vi "Main.vi"() -> ()   [LabVIEW 2020, in "S7.lvlib"]
doc: "This template is based off of the Queued Message Handler design pattern and the Queued Message Handler project template that ships with LabVIEW.\n\nThe main difference is that the queue is private to this module and communication between modules is performed via Broadcast and Request events.\n\nRequest events are wrapped in public API methods and are handled in the Event Handling Loop (EHL) of this VI. Any module can register for Broadcast events sent by this module. The EHL generates messages based on user interface actions.\n\nThe Message Handling Loop (MHL) processes messages generated by the EHL, or by other messages. The messages are string values, so new messages can be added easily to the Message Cases case structure in the MHL. Each message cluster can also provide an optional value for Message Data, which is a variant that can be converted to whatever message-specific data is required.\n_____\nBased on Delacor QMH Project Template 4.1.0.59."
uses:
  S7.lvlib
  <vilib>/Delacor/Delacor QMH/Libraries/Module Admin_class/Delacor_lib_QMH_Module Admin.lvclass
  Module Data--cluster.ctl
  <vilib>/Delacor/Delacor QMH/Libraries/Message Queue_class/Delacor_lib_QMH_Message Queue.lvclass/Delacor_lib_QMH_Message Queue.ctl
  Stop Argument--cluster.ctl
  <vilib>/Delacor/Delacor QMH/Libraries/Module Admin_class/Delacor_lib_QMH_Module Admin.lvclass/Delacor_lib_QMH_Module Admin.ctl
  Init S7 Link Argument--cluster.ctl
  Close S7 Link Argument--cluster.ctl
  Read_Data Argument--cluster.ctl
  Read_Data (Reply Payload)--cluster.ctl
  Write_Data Argument--cluster.ctl
  Write_Data (Reply Payload)--cluster.ctl
  <vilib>/Utility/miscctls.llb/LVPointTypeDef.ctl
  <vilib>/Delacor/Delacor QMH/Libraries/Message Queue_class/Delacor_lib_QMH_Enqueue Message (Single).vi
  <vilib>/Delacor/Delacor QMH/Libraries/Module Admin_class/Delacor_lib_QMH_Get External Launch.vi
  <vilib>/Utility/error.llb/Error Cluster From Error Code.vi
  <vilib>/ErrorRing/Error Ring.xnode
  <vilib>/Delacor/Delacor QMH/Libraries/Message Queue_class/Delacor_lib_QMH_Message Queue.lvclass
panel:
  out "S7 Link":refnum<k5>
  in  "Simulate MHL Error":bool
  in  "Simulate EHL Error":bool
  out "error out":errorcluster
  in  "Module Admin":refnum<class "Delacor_lib_QMH_Module Admin.lvclass">
  out "Status":string
  # "Other QMH Modules communicate with this Module via its Public API (wrappers for its Request Events).\n\nThis Module communicates with other Modules via its Broadcast Events.\nAny module that wants to get these messages, just registers for this module's Broadcast events."
  # "This template is for the Delacor Modified Queued Message Handler design pattern.\n\nSee the block diagram for more information on how to use this template."
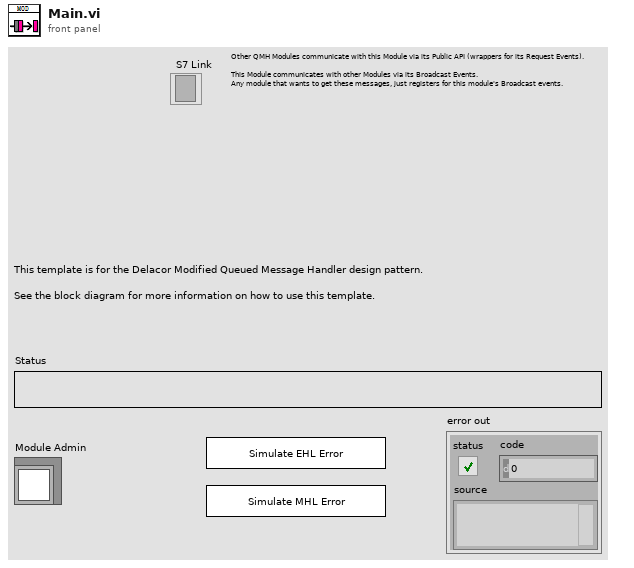
[diagram p1: front panel]
types:
  T1 = typedef "S7.lvlib/Request Events--cluster.ctl" = cluster{"Stop Module":refnum<user-event>, "Show Panel":refnum<user-event>, "Hide Panel":refnum<user-event>, "Get Module Execution Status":refnum<user-event>, "Show Diagram":refnum<user-event>, "S7_Open":refnum<user-event>, "Init S7 Link":refnum<user-event>, "Close S7 Link":refnum<user-event>, "Read_Data":refnum<user-event>, "Write_Data":refnum<user-event>}
  T2 = typedef "S7.lvlib/Module Data--cluster.ctl" = cluster{"Status":string}
  T3 = enum32{"invalid lock state", "Not Locked", "Locked (No Password)", "Password-protected"}
  T4 = typedef "S7.lvlib/Stop Argument--cluster.ctl" = cluster{"Origin":string, "Exit via Stop Module Req?":bool, "Wait for Module to stop?":bool}
  T5 = typedef "S7.lvlib/Init S7 Link Argument--cluster.ctl" = cluster{"IP":string, "超时":i32}
  T6 = typedef "S7.lvlib/Close S7 Link Argument--cluster.ctl" = cluster{"布尔":bool}
  T7 = typedef "S7.lvlib/Read_Data Argument--cluster.ctl" = cluster{"DB #":u16, "起始地址":u32, "寄存器类型":u8, "读取长度":u16, "数据类型":u16, "Wait Notifier":refnum<notifier>, "wait for reply":bool}
  T8 = typedef "S7.lvlib/Write_Data Argument--cluster.ctl" = cluster{"写入数据":u32, "DB #":u16, "写入地址":u32, "寄存器类型":u8, "数据类型":u16, "Wait Notifier":refnum<notifier>, "wait for reply":bool}
  T9 = typedef "LVPointTypeDef.ctl" = cluster{"Horizontal":i16, "Vertical":i16}
  T10 = enum32{"Invalid", "Standard", "Closed", "Hidden", "Minimized", "Maximized"}
  T11 = typedef "S7.lvlib/Read_Data (Reply Payload)--cluster.ctl" = cluster{"读取成功":bool, "数据":u32[], "Read_Data_error":errorcluster}
  T12 = typedef "S7.lvlib/Write_Data (Reply Payload)--cluster.ctl" = cluster{"写入成功":bool, "Write_Data_error":errorcluster}
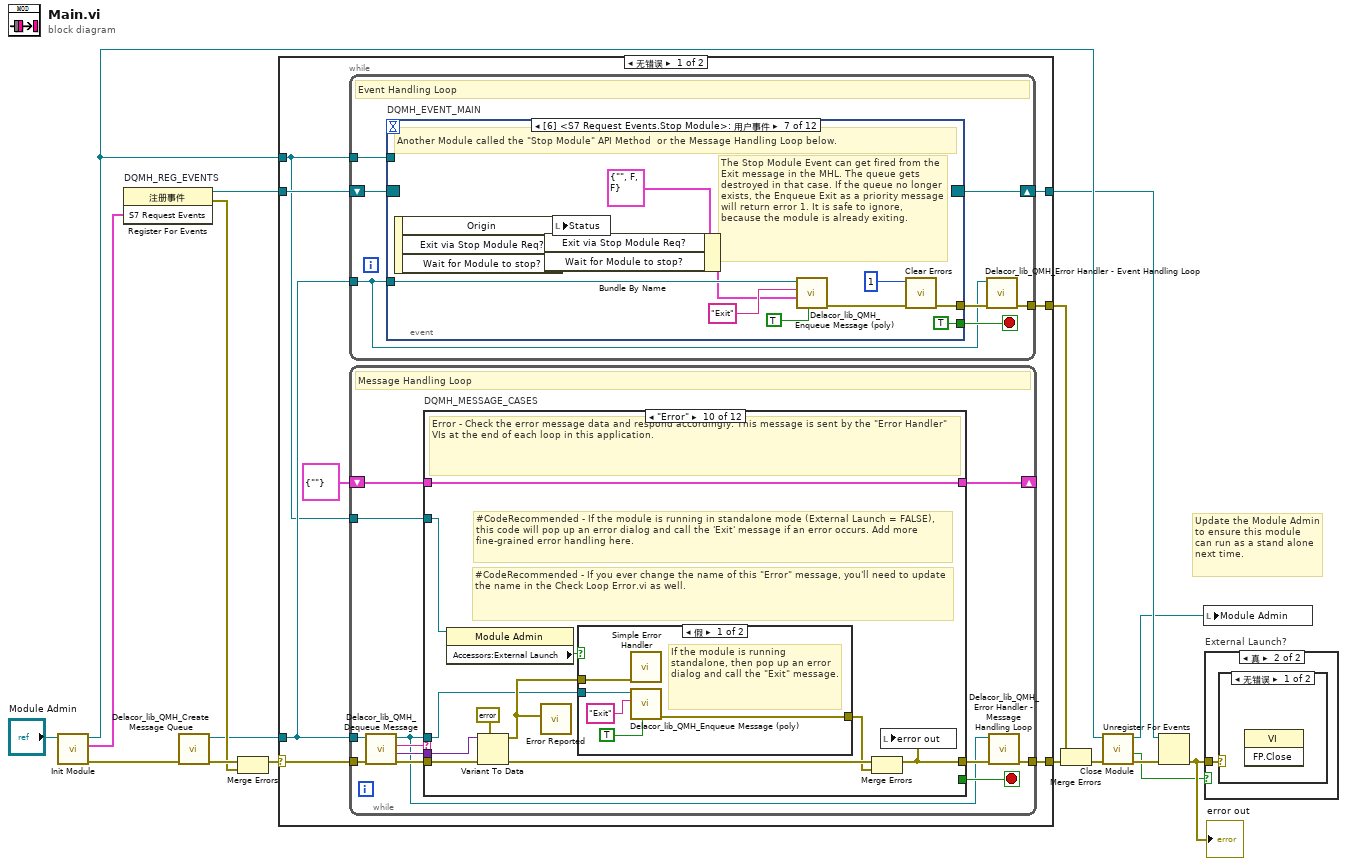
[diagram p0: block diagram]
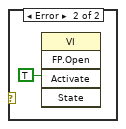
[diagram p3: hidden frame]
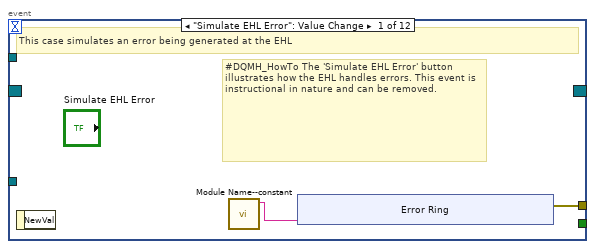
[diagram p4: hidden frame]
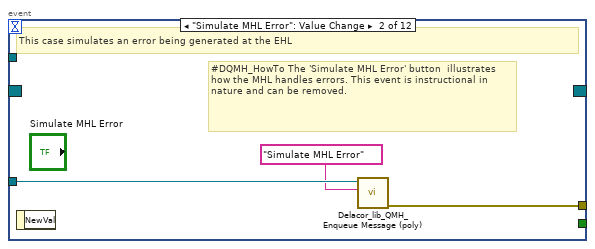
[diagram p5: hidden frame]
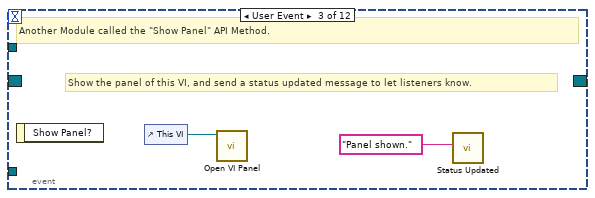
[diagram p6: hidden frame]
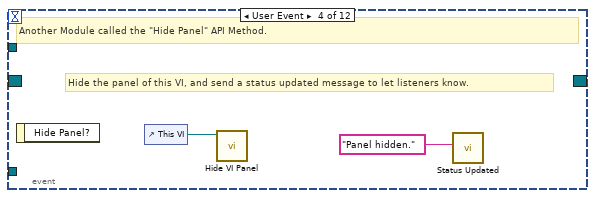
[diagram p7: hidden frame]
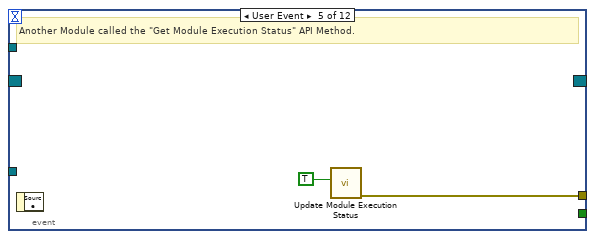
[diagram p8: hidden frame]
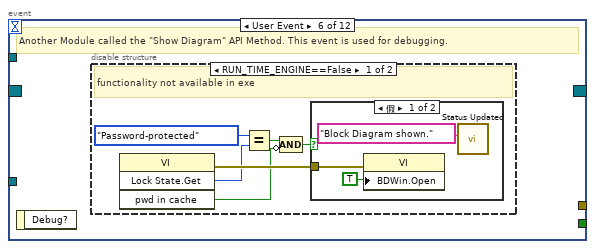
[diagram p9: hidden frame]
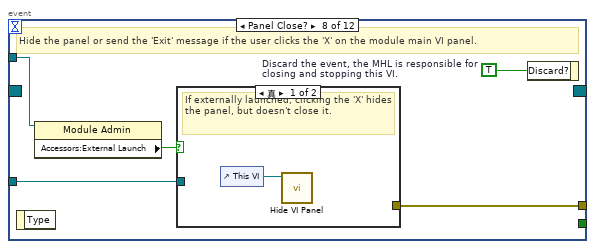
[diagram p12: hidden frame]
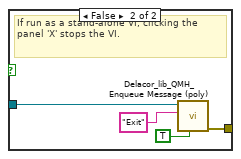
[diagram p13: hidden frame]
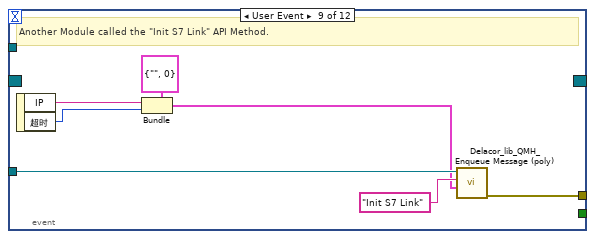
[diagram p14: hidden frame]
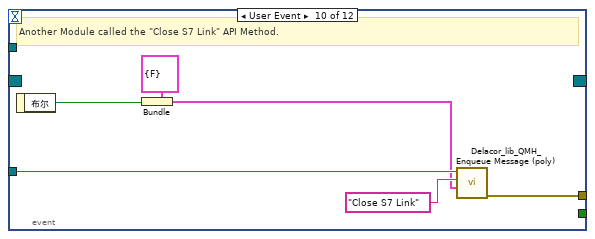
[diagram p15: hidden frame]
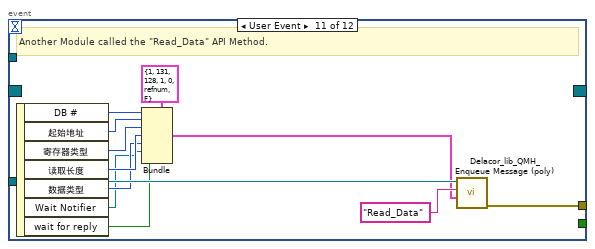
[diagram p16: hidden frame]
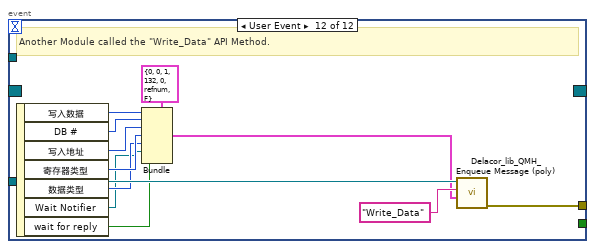
[diagram p17: hidden frame]
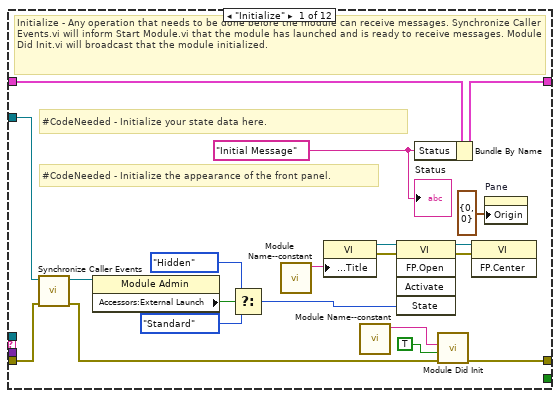
[diagram p18: hidden frame]
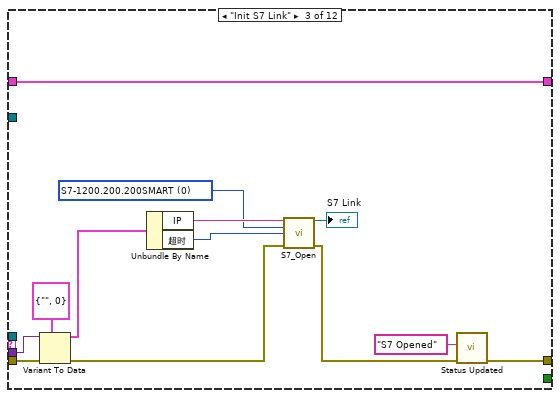
[diagram p20: hidden frame]
diagram:
  # "Update the Module Admin to ensure this module can run as a stand alone next time."
  n1 = call "Init Module.vi"("Singleton Module Admin in"="Module Admin") -> ("error out"=w16:errorcluster, "S7 Request Events"=w5:T1, "Singleton Module Admin out"=w8:refnum<class "Delacor_lib_QMH_Module Admin.lvclass">)  [unwired: 8 in]
  n2 = register-events "DQMH_REG_EVENTS"(w5) -> (reference out=w6:refnum<event-registration>, error out=w9:errorcluster)  [unwired: 2 in]
  n3 = call <vilib>:"Delacor_lib_QMH_Create Message Queue.vi"("error in"=w16) -> ("error out"=w11:errorcluster, "Message Queue"=w4:refnum<class "Delacor_lib_QMH_Message Queue.lvclass">)  [unwired: 9 in]
  n4 = Merge Errors(w11, w9) -> (w10:errorcluster)
  n5 = case shown="无错误" w10 {
    selector: w10 -> [w23 w290]
    tunnel: [w25 w290] -> w17
    tunnel: [w22 w287] -> w7
    tunnel: w6 -> [w20 w287]
    tunnel: w4 -> [w19 _]
    tunnel: [w24 _] -> w14
    tunnel: w8 -> [w18 w283]
    frame No Error {
      n6 = while {
        tunnel: w19 -> [w26]
        shift-right: [w29] -> w22
        shift-left: w20 -> [w30]
        tunnel: [w31] -> w24
        tunnel: w18 -> [w27]
        stop <- w28 stop-if-true
        # "Event Handling Loop"
        n7 = event "DQMH_EVENT_MAIN" shown="[6] <S7 Request Events.Stop Module>: 用户事件" {
          selector: w30 -> [_ _ _ _ _ _ _ _ _ _ _ _]
          dyn-events: [_ _ _ _ _ _ _ _ _ _ _ _] -> w29
          timeout: _ -> [_ _ _ _ _ _ _ _ _ _ _ _]
          tunnel: [_ _ _ _ _ _ TRUE ("Discard?") _ _ _ _ _] -> w28
          tunnel: w26 -> [_ w43 _ _ _ _ w67 w74 w88 w94 w106 w118]
          tunnel: [w34 w44 _ _ w50 _ w70 w76 w82 w89 w95 w107] -> w32
          tunnel: w27 -> [_ _ _ _ _ _ _ w73 _ _ _ _]
          event "Simulate EHL Error": Value Change {
            # "#DQMH_HowTo The 'Simulate EHL Error' button  illustrates how the EHL handles errors. This event is instructional in nature and can be removed."
            # "This case simulates an error being generated at the EHL"
            n8 = event-data() -> ()  [unwired: 1 in, 1 out]
            n9 = call "Module Name--constant.vi"() -> ("Module Name"=w33:string)  [unwired: 11 in]
            n10 = xnode "Error Ring"("参数 0"=w33) -> ("错误输出"=w34:errorcluster)
          }
          event "Simulate MHL Error": Value Change {
            # "#DQMH_HowTo The 'Simulate MHL Error' button  illustrates how the MHL handles errors. This event is instructional in nature and can be removed."
            # "This case simulates an error being generated at the EHL"
            n11 = event-data() -> ()  [unwired: 1 in, 1 out]
            n12 = call-poly <vilib>:"Delacor_lib_QMH_Enqueue Message (poly).vi"("Message"="Simulate MHL Error", "Message Queue in"=w43) -> ("error out"=w44:errorcluster)  [unwired: 8 in, 1 out]
          }
          event User Event {
            # "Show the panel of this VI, and send a status updated message to let listeners know."
            # "Another Module called the \"Show Panel\" API Method."
            n13 = event-data() -> ()  [unwired: 1 in, 1 out]
            n14 = control-ref of="This VI"() -> (w46:refnum<vi>)
            n15 = call "Open VI Panel.vi"("VI"=w46) -> ()  [unwired: 10 in, 1 out]
            n16 = call "Status Updated.vi"("Status"="Panel shown." ("format string")) -> ()  [unwired: 10 in, 1 out]
          }
          event User Event {
            # "Hide the panel of this VI, and send a status updated message to let listeners know."
            # "Another Module called the \"Hide Panel\" API Method."
            n17 = event-data() -> ()  [unwired: 1 in, 1 out]
            n18 = control-ref of="This VI"() -> (w48:refnum<vi>)
            n19 = call "Hide VI Panel.vi"("VI"=w48) -> ()  [unwired: 10 in, 1 out]
            n20 = call "Status Updated.vi"("Status"="Panel hidden." ("format string")) -> ()  [unwired: 10 in, 1 out]
          }
          event User Event {
            # "Another Module called the \"Get Module Execution Status\" API Method."
            n21 = event-data() -> ()  [unwired: 1 in, 1 out]
            n22 = call "Update Module Execution Status.vi"("Running?"=TRUE) -> ("error out"=w50:errorcluster)  [unwired: 10 in]
          }
          event User Event {
            # "Another Module called the \"Show Diagram\" API Method. This event is used for debugging."
            n23 = event-data() -> ()  [unwired: 1 in, 1 out]
            n24 = disable-structure shown="RUN_TIME_ENGINE==False" {
              frame condition #0 (active) {
                # "functionality not available in exe"
                n25 = invoke class="VI" method="Lock State.Get"() -> (error out=w56:errorcluster, "Get Lock State"=w55:T3, "pwd in cache"=w52:bool)  [unwired: 4 in, 1 out]
                n26 = Equal?(x=T3."Password-protected", y=w55) -> (x = y?=w53:bool)
                n27 = Compound Arithmetic op=AND(w53, invert w52) -> (w51:bool)
                n28 = case "条件结构" shown="假" w51 {
                  tunnel: w56 -> [w59 _]
                  frame False {
                    n29 = property class="VI"(error in=w59, "BDWin.Open"=TRUE ("Block Diagram Window:Open")) -> ()  [unwired: 1 in, 2 out]
                    n30 = call "Status Updated.vi"("Status"="Block Diagram shown." ("format string")) -> ()  [unwired: 10 in, 1 out]
                  }
                  frame True {
                    # "Password-protected VI, and the password is not in the cache. Do not show the diagram."
                  }
                }
              }
              frame condition #1 {
              }
            }
          }
          event User Event {
            # "The Stop Module Event can get fired from the Exit message in the MHL. The queue gets destroyed in that case. If the queue no longer exists, the Enqueue Exit as a priority message will return error 1. It is safe to ignore, because the module is already exiting."
            # "Another Module called the \"Stop Module\" API Method  or the Message Handling Loop below."
            n31 = event-data() -> ("Origin"=w66:string, "Exit via Stop Module Req?"=w62:bool, "Wait for Module to stop?"=w61:bool)  [unwired: 1 in]
            n32 = Bundle By Name(cluster=T4 {"Origin"="", "Exit via Stop Module Req?"=FALSE, "Wait for Module to stop?"=FALSE} ("Stop Argument"), "Exit via Stop Module Req?"=w62, "Wait for Module to stop?"=w61) -> (w60:T4)
            n33 = local write "Status"(w66) -> ()
            n34 = call-poly <vilib>:"Delacor_lib_QMH_Enqueue Message (poly).vi"("Priority Message? (F)"=TRUE, "Message Data"=w60, "Message"="Exit", "Message Queue in"=w67) -> ("error out"=w71:errorcluster)  [unwired: 6 in, 1 out]
            n35 = call <vilib>:"Clear Errors.vi"("error in (no error)"=w71, "specific error code to clear (0: all)"=1) -> ("error out"=w70:errorcluster)  [unwired: 4 in, 1 out]
          }
          event Panel Close? {
            w75 = TRUE  # Discard the event, the MHL is responsible for closing and stopping this VI.
            # "Hide the panel or send the 'Exit' message if the user clicks the 'X' on the module main VI panel."
            n36 = event-data() -> ()  [unwired: 1 in, 1 out]
            n37 = property class="Module Admin"(reference=w73) -> ("Accessors:External Launch"=w72:bool)  [unwired: 1 in, 2 out]
            n38 = case "条件结构" shown="真" w72 {
              tunnel: w74 -> [_ w80]
              tunnel: [_ w81] -> w76
              frame True {
                # "If externally launched, clicking the 'X' hides the panel, but doesn't close it."
                n39 = control-ref of="This VI"() -> (w77:refnum<vi>)
                n40 = call "Hide VI Panel.vi"("VI"=w77) -> ()  [unwired: 10 in, 1 out]
              }
              frame False {
                # "If run as a stand-alone VI, clicking the panel 'X' stops the VI."
                n41 = call-poly <vilib>:"Delacor_lib_QMH_Enqueue Message (poly).vi"("Priority Message? (F)"=TRUE, "Message"="Exit", "Message Queue in"=w80) -> ("error out"=w81:errorcluster)  [unwired: 7 in, 1 out]
              }
            }
            n42 = event-data("Discard?"=w75) -> ()  [unwired: 1 in, 1 out]
          }
          event User Event {
            # "Another Module called the \"Init S7 Link\" API Method."
            n43 = event-data() -> ("IP"=w84:string, "超时"=w83:i32)  [unwired: 1 in]
            n44 = Bundle(cluster=T5 {"IP"="", "超时"=0} ("Init S7 Link Argument"), "IP"=w84, "超时"=w83) -> (w85:T5)
            n45 = call-poly <vilib>:"Delacor_lib_QMH_Enqueue Message (poly).vi"("Message Data"=w85, "Message"="Init S7 Link", "Message Queue in"=w88) -> ("error out"=w82:errorcluster)  [unwired: 7 in, 1 out]
          }
          event User Event {
            # "Another Module called the \"Close S7 Link\" API Method."
            n46 = event-data() -> ("布尔"=w90:bool)  [unwired: 1 in]
            n47 = Bundle(cluster=T6 {"布尔"=FALSE} ("Close S7 Link Argument"), "布尔"=w90) -> (w91:T6)
            n48 = call-poly <vilib>:"Delacor_lib_QMH_Enqueue Message (poly).vi"("Message Data"=w91, "Message"="Close S7 Link", "Message Queue in"=w94) -> ("error out"=w89:errorcluster)  [unwired: 7 in, 1 out]
          }
          event User Event {
            # "Another Module called the \"Read_Data\" API Method."
            n49 = event-data() -> ("DB #"=w102:u16, "起始地址"=w101:u32, "寄存器类型"=w100:u8, "读取长度"=w99:u16, "数据类型"=w98:u16, "Wait Notifier"=w97:refnum<notifier>, "wait for reply"=w96:bool)  [unwired: 1 in]
            n50 = Bundle(cluster=T7 {"DB #"=1, "起始地址"=131, "寄存器类型"=128, "读取长度"=1, "数据类型"=0, "Wait Notifier"=refnum, "wait for reply"=FALSE} ("Read_Data Argument"), "DB #"=w102, "起始地址"=w101, "寄存器类型"=w100, "读取长度"=w99, "数据类型"=w98, "Wait Notifier"=w97, "wait for reply"=w96) -> (w103:T7)
            n51 = call-poly <vilib>:"Delacor_lib_QMH_Enqueue Message (poly).vi"("Message Data"=w103, "Message"="Read_Data", "Message Queue in"=w106) -> ("error out"=w95:errorcluster)  [unwired: 7 in, 1 out]
          }
          event User Event {
            # "Another Module called the \"Write_Data\" API Method."
            n52 = event-data() -> ("写入数据"=w114:u32, "DB #"=w113:u16, "写入地址"=w112:u32, "寄存器类型"=w111:u8, "数据类型"=w110:u16, "Wait Notifier"=w109:refnum<notifier>, "wait for reply"=w108:bool)  [unwired: 1 in]
            n53 = Bundle(cluster=T8 {"写入数据"=0, "DB #"=0, "写入地址"=1, "寄存器类型"=132, "数据类型"=0, "Wait Notifier"=refnum, "wait for reply"=FALSE} ("Write_Data Argument"), "写入数据"=w114, "DB #"=w113, "写入地址"=w112, "寄存器类型"=w111, "数据类型"=w110, "Wait Notifier"=w109, "wait for reply"=w108) -> (w115:T8)
            n54 = call-poly <vilib>:"Delacor_lib_QMH_Enqueue Message (poly).vi"("Message Data"=w115, "Message"="Write_Data", "Message Queue in"=w118) -> ("error out"=w107:errorcluster)  [unwired: 7 in, 1 out]
          }
        }
        n55 = call-dynamic "Delacor_lib_QMH_Error Handler - Event Handling Loop.vi"("error in"=w32, "Message Queue in"=w26) -> ("dup error in"=w31:errorcluster)  [unwired: 8 in, 1 out]
      }
      n56 = while {
        tunnel: w19 -> [w121]
        shift-right: [w125] -> _
        shift-left: T2 {"Status"=""} ("Data Cluster") -> [w126]
        tunnel: w23 -> [w129]
        tunnel: [w127] -> w25
        tunnel: w18 -> [w119]
        stop <- w124 stop-if-true
        # "Message Handling Loop"
        n57 = call-dynamic "Delacor_lib_QMH_Dequeue Message.vi"("error in"=w129, "Message Queue in"=w121) -> ("error out"=w128:errorcluster, "Message Data"=w122:variant, "Message"=w123:string, "Message Queue out"=w120:refnum<class "Delacor_lib_QMH_Message Queue.lvclass">)  [unwired: 6 in]
        n58 = case "DQMH_MESSAGE_CASES" shown="\"Error\"" w123 {
          selector: w123 -> [_ _ _ _ _ _ _ _ _ _ _ w270]
          tunnel: w120 -> [_ _ _ _ _ _ _ _ _ w240 w262 _]
          tunnel: w128 -> [w148 w152 w165 w173 w197 w218 w223 w225 w230 w247 w268 w272]
          tunnel: [w146 w152 w154 w166 w188 w209 w222 w225 w229 w243 w265 w273] -> w130
          tunnel: w126 -> [w137 w151 w164 w172 w196 w217 w221 w224 w227 w242 w261 w271]
          tunnel: [w136 w151 w164 w172 w196 w217 w221 w224 w227 w242 w261 w271] -> w125
          tunnel: [_ _ _ _ _ _ _ _ _ _ w260 _] -> w124
          tunnel: w122 -> [_ _ w163 w171 w195 w216 _ _ _ w241 w259 _]
          tunnel: w119 -> [w138 _ _ _ _ _ _ _ _ w239 w254 _]
          frame "Initialize" {
            w131 = "Initial Message" ("Initial Message")
            # "#CodeNeeded - Initialize the appearance of the front panel."
            # "#CodeNeeded - Initialize your state data here."
            # "Initialize - Any operation that needs to be done before the module can receive messages. Synchronize Caller Events.vi will inform Start Module.vi that the module has launched and is ready to receive messages. Module Did Init.vi will broadcast that the module initialized."
            n59 = call "Synchronize Caller Events.vi"("error in (no error)"=w148, "Singleton Module Admin in"=w138) -> ("error out"=w147:errorcluster, "Singleton Module Admin out"=w133:refnum<class "Delacor_lib_QMH_Module Admin.lvclass">)  [unwired: 8 in]
            n60 = property class="Module Admin"(reference=w133) -> ("Accessors:External Launch"=w142:bool)  [unwired: 1 in, 2 out]
            n61 = Select(t=T10."Hidden" ("State"), s=w142, f=T10."Standard" ("State")) -> (s? t:f=w139:T10)
            n62 = call "Module Name--constant.vi"() -> ("Module Name"=w145:string)  [unwired: 11 in]
            n63 = property class="VI"("Front Panel.Title"=w145) -> (reference out=w144:refnum<vi>, error out=w150:errorcluster)  [unwired: 2 in]
            n64 = call "Module Name--constant.vi"() -> ("Module Name"=w134:string)  [unwired: 11 in]
            n65 = invoke class="VI" method="FP.Open"(reference=w144, error in=w150, "State"=w139) -> (reference out=w143:refnum<vi>, error out=w149:errorcluster)  [unwired: 2 in, 3 out]
            n66 = Bundle By Name(cluster=w137, "Status"=w131) -> (w136:T2)
            n67 = call "Module Did Init.vi"("error in (no error)"=w147, "Initialized?"=TRUE, "Origin"=w134) -> ("error out"=w146:errorcluster)  [unwired: 8 in]
            n68 = invoke class="VI" method="FP.Center"(reference=w143, error in=w149) -> ()  [unwired: 1 in, 3 out]
            n69 = property on="Pane" class="Pane"("Origin"=T9 {"Horizontal"=0, "Vertical"=0}) -> ()  [unwired: 2 in, 2 out]
            "Status" <- w131
          }
          frame "--- Module Specific ---" {
            # "Separator -- The following cases handle messages specific to this Module."
          }
          frame "Init S7 Link" {
            w159 = u8 0 items=["S7-1200.200.200SMART"=0, "S7-300"=2, "S7-400"=3] ("PLC 系列")
            n70 = Variant To Data(error in=w165, type=T5 {"IP"="", "超时"=0} ("Init S7 Link Argument"), Variant=w163) -> (data=w161:T5, error out=w156:errorcluster)
            n71 = Unbundle By Name(w161) -> ("IP"=w160:string, "超时"=w158:i32)
            n72 = call "S7_Open.vi"("IP 地址"=w160, "PLC 系列"=w159, "超时（MS）"=w158, "error in"=w156) -> ("TCP"=→"S7 Link":refnum<k5>, "error out"=w155:errorcluster)  [unwired: 9 in, 1 out]
            n73 = call "Status Updated.vi"("error in (no error)"=w155, "Status"="S7 Opened") -> ("error out"=w154:errorcluster)  [unwired: 9 in]
          }
          frame "Close S7 Link" {
            n74 = Variant To Data(error in=w173, type=T6 {"布尔"=FALSE} ("Close S7 Link Argument"), Variant=w171) -> (data=w169:T6, error out=w167:errorcluster)
            n75 = Unbundle By Name(w169) -> ("布尔"=w168:bool)
            n76 = case shown="真" w168 {
              tunnel: w167 -> [w174 w176]
              tunnel: [w174 w175] -> w166
              frame False {
              }
              frame True {
                n77 = local read "S7 Link"() -> (w177:refnum<k5>)
                n78 = call "S7_Close.vi"("error in"=w176, "TCP Connection Ref"=w177) -> ("error out"=w175:errorcluster)  [unwired: 9 in]
              }
            }
          }
          frame "Read_Data" {
            n79 = Variant To Data(error in=w197, type=T7 {"DB #"=1, "起始地址"=131, "寄存器类型"=128, "读取长度"=1, "数据类型"=0, "Wait Notifier"=refnum, "wait for reply"=FALSE} ("Read_Data Argument"), Variant=w195) -> (data=w193:T7, error out=w180:errorcluster)
            n80 = local read "S7 Link"() -> (w187:refnum<k5>)
            n81 = Unbundle By Name(w193) -> ("读取长度"=w186:u16, "DB #"=w185:u16, "寄存器类型"=w184:u8, "起始地址"=w183:u32, "数据类型"=w182:u16, "Wait Notifier"=w192:refnum<notifier>, "wait for reply"=w191:bool)
            n82 = call "S7_Read.vi"("TCP"=w187, "DB #"=w185, "读取长度"=w186, "寄存器类型"=w184, "起始地址"=w183, "数据类型"=w182, "error in"=w180) -> ("数据"=w179:u32[], "读取成功"=w178:bool, "error out"=w181:errorcluster)  [unwired: 5 in, 1 out]
            n83 = Merge Errors(w180, w181) -> (w188:errorcluster)
            n84 = Bundle By Name(cluster=T11 {"读取成功"=FALSE, "数据"=[], "Read_Data_error"={"status"=FALSE, "code"=0, "source"=""}} ("Read_Data (Reply Payload)"), "读取成功"=w178, "数据"=w179, "Read_Data_error"=w181) -> (w190:T11)
            n85 = case shown="真" w191 {
              tunnel: w192 -> [_ w199]
              tunnel: w190 -> [_ w198]
              frame False {
              }
              frame True {
                n86 = Send Notification(notification=w198, notifier=w199) -> ()  [unwired: 1 in, 2 out]
              }
            }
          }
          frame "Write_Data" {
            n87 = Variant To Data(error in=w218, type=T8 {"写入数据"=0, "DB #"=0, "写入地址"=1, "寄存器类型"=132, "数据类型"=0, "Wait Notifier"=refnum, "wait for reply"=FALSE} ("Write_Data Argument"), Variant=w216) -> (data=w214:T8, error out=w202:errorcluster)
            n88 = local read "S7 Link"() -> (w200:refnum<k5>)
            n89 = Unbundle By Name(w214) -> ("DB #"=w208:u16, "寄存器类型"=w207:u8, "写入地址"=w206:u32, "数据类型"=w205:u16, "写入数据"=w204:u32, "Wait Notifier"=w213:refnum<notifier>, "wait for reply"=w212:bool)
            n90 = call "S7_Write.vi"("TCP"=w200, "寄存器类型"=w207, "DB #"=w208, "写入地址"=w206, "数据类型"=w205, "写入数据"=w204, "error in"=w202) -> ("写入成功"=w203:bool, "error out"=w201:errorcluster)  [unwired: 6 in, 1 out]
            n91 = Merge Errors(w202, w201) -> (w209:errorcluster)
            n92 = Bundle By Name(cluster=T12 {"写入成功"=FALSE, "Write_Data_error"={"status"=FALSE, "code"=0, "source"=""}} ("Write_Data (Reply Payload)"), "写入成功"=w203, "Write_Data_error"=w201) -> (w211:T12)
            n93 = case shown="真" w212 {
              tunnel: w213 -> [_ w220]
              tunnel: w211 -> [_ w219]
              frame False {
              }
              frame True {
                n94 = Send Notification(notification=w219, notifier=w220) -> ()  [unwired: 1 in, 2 out]
              }
            }
          }
          frame "---Copy This Frame---" {
            # "Duplicate this frame when creating new messages.  Change this comment in the duplicated frame to describe this message."
            n95 = Merge Errors(w223) -> (w222:errorcluster)
          }
          frame "--- Exit and Error Handling---" {
            # "Separator - The following cases handle errors and exit messages."
          }
          frame "Simulate MHL Error" {
            # "#DQMH_HowTo The 'Simulate MHL Error' button  illustrates how the MHL handles errors. This event is instructional in nature and can be removed."
            # "Simulate an error occurring at the MHL"
            n96 = call "Module Name--constant.vi"() -> ("Module Name"=w226:string)  [unwired: 11 in]
            n97 = xnode "Error Ring"("参数 0"=w226) -> ("错误输出"=w228:errorcluster)
            n98 = Merge Errors(w230, w228) -> (w229:errorcluster)
          }
          frame "Error" {
            # "#CodeRecommended - If you ever change the name of this \"Error\" message, you'll need to update the name in the Check Loop Error.vi as well."
            # "#CodeRecommended - If the module is running in standalone mode (External Launch = FALSE), this code will pop up an error dialog and call the 'Exit' message if an error occurs. Add more fine-grained error handling here."
            # "Error - Check the error message data and respond accordingly. This message is sent by the \"Error Handler\" VIs at the end of each loop in this application."
            n99 = property class="Module Admin"(reference=w239) -> ("Accessors:External Launch"=w238:bool)  [unwired: 1 in, 2 out]
            n100 = Variant To Data(error in=w247, type=errorcluster {"status"=FALSE, "code"=0, "source"=""} ("error constant"), Variant=w241) -> (data=w248:errorcluster, error out=w245:errorcluster)
            n101 = call "Error Reported.vi"("Error"=w248) -> ()  [unwired: 10 in, 1 out]
            n102 = case shown="假" w238 {
              tunnel: [w253 _] -> w244
              tunnel: w240 -> [w251 _]
              tunnel: w248 -> [w252 _]
              frame False {
                # "If the module is running standalone, then pop up an error dialog and call the \"Exit\" message."
                n103 = call <vilib>:"Simple Error Handler.vi"("error in (no error)"=w252) -> ()  [unwired: 4 in, 5 out]
                n104 = call-poly <vilib>:"Delacor_lib_QMH_Enqueue Message (poly).vi"("Priority Message? (F)"=TRUE, "Message"="Exit", "Message Queue in"=w251) -> ("error out"=w253:errorcluster)  [unwired: 7 in, 1 out]
              }
              frame True {
                # "If the module was launched externally, calling the Error Reported broadcast VI is the only action performed by the \"Error\" message. The module's caller can then process the error appropriately."
              }
            }
            n105 = Merge Errors(w245, w244) -> (w243:errorcluster)
            n106 = local write "error out"(w243) -> ()
          }
          frame "Exit" {
            w258 = 91  # 91: not all Exit messages will have an argument
            w260 = TRUE  # Stop the VI
            # "Release the message queue reference"
            # "#CodeNeeded - Add any required cleanup code here"
            # "Exit - Exit the application."
            n107 = Variant To Data(error in=w268, type=T4 {"Origin"="", "Exit via Stop Module Req?"=FALSE, "Wait for Module to stop?"=FALSE} ("Stop Argument"), Variant=w259) -> (data=w256:T4, error out=w264:errorcluster)
            n108 = call <vilib>:"Clear Errors.vi"("error in (no error)"=w264, "specific error code to clear (0: all)"=w258) -> ("error out"=w267:errorcluster)  [unwired: 4 in, 1 out]
            n109 = control-ref of="This VI"() -> (w255:refnum<vi>)
            n110 = call-dynamic "Delacor_lib_QMH_Release Message Queue.vi"("error in"=w267, "Message Queue"=w262) -> ("error out"=w266:errorcluster)  [unwired: 9 in]
            n111 = call "Handle Exit.vi"("Stop Argument"=w256, "Admin in"=w254, "VI reference"=w255) -> ("error out"=w263:errorcluster)  [unwired: 7 in, 1 out]
            n112 = Merge Errors(w266, w263) -> (w265:errorcluster)
          }
          frame Default {
            # "'Default' case only runs if there is a message that isn't defined in any of the other cases.  Output a programming error."
            n113 = call "Module Name--constant.vi"() -> ("Module Name"=w269:string)  [unwired: 11 in]
            n114 = xnode "Error Ring"("参数 0"=w270, "参数 1"=w269) -> ("错误输出"=w274:errorcluster)
            n115 = Merge Errors(w272, w274) -> (w273:errorcluster)
          }
        }
        n116 = call-dynamic "Delacor_lib_QMH_Error Handler - Message Handling Loop.vi"("error in"=w130, "Message Queue in"=w120) -> ("dup error in"=w127:errorcluster)  [unwired: 8 in, 1 out]
      }
    }
    frame Error {
      # "Synchronize Caller Events.vi will inform Start Module.vi that the module has launched and will let the code calling Start Module.vi register for broadcasts and would permit the caller receive the broadcast that an error occurred at launch time."
      n117 = call "Synchronize Caller Events.vi"("Singleton Module Admin in"=w283) -> ("error out"=w288:errorcluster)  [unwired: 9 in, 1 out]
      n118 = call "Module Name--constant.vi"() -> ("Module Name"=w286:string)  [unwired: 11 in]
      n119 = Format Into String(format string="An error occurred during initialization. %s is no longer running.", w286) -> (resulting string=w284:string)  [unwired: 2 in, 1 out]
      n120 = Merge Errors(w290, w288) -> (w289:errorcluster)
      n121 = call "Error Reported.vi"("Additional Information"=w284, "Error"=w289) -> ()  [unwired: 9 in, 1 out]
    }
  }
  n122 = Merge Errors(w14, w17) -> (w13:errorcluster)
  n123 = call "Close Module.vi"("error in (no error)"=w13, "Module Admin in"=w8) -> ("error out"=w15:errorcluster, "External Launch"=w1:bool, "Module Admin out"=w2:refnum<class "Delacor_lib_QMH_Module Admin.lvclass">)  [unwired: 7 in]
  n124 = Unregister For Events(event registration refnum=w7, error in=w15) -> (error out=w12:errorcluster)
  "error out" <- w12
  n125 = local write "Module Admin"(w2) -> ()
  n126 = case "External Launch?" shown="真" w1 {
    tunnel: w12 -> [_ w291]
    frame False {
    }
    frame True {
      n127 = case "条件结构" shown="无错误" w291 {
        frame No Error {
          n128 = invoke class="VI" method="FP.Close"() -> ()  [unwired: 3 in, 3 out]
        }
        frame Error {
          n129 = invoke class="VI" method="FP.Open"("Activate"=TRUE ("Activate?")) -> ()  [unwired: 4 in, 5 out]
        }
      }
    }
  }
